vi "respond to response.vi"(8 "error in (no error)":errorcluster caption="Fehler (Eingang, kein Fehler)", 10 "?":T1={"commandlist"="", "line"=0, "last response"="", "timeout"=0, "wait"=0, "erfolgreich"=FALSE, "next state"=enum."init", "Zustand"=enum."starting", "manual Test"=FALSE}, 11 "Surge Eingang":refnum<class "Surge.lvclass"> caption="DNL_LabVIEW Object in") -> (0 "error out":errorcluster caption="Fehler (Ausgang)", 1 "read again?":bool, 2 "?":T1={"commandlist"="", "line"=0, "last response"="", "timeout"=0, "wait"=0, "erfolgreich"=FALSE, "next state"=enum."init", "Zustand"=enum."starting", "manual Test"=FALSE}, 3 "Surge Ausgang":refnum<class "Surge.lvclass"> caption="DNL_LabVIEW Object out")   [LabVIEW 2013, in "Surge.lvclass"]
uses:
  Surge.lvclass
  Main/controls/TestData.ctl
  Main/controls/TestStates.ctl
  Main/controls/generalTestStates.ctl
  lib/EMV-Test.lvlib
panel:
  out "cmdl":string
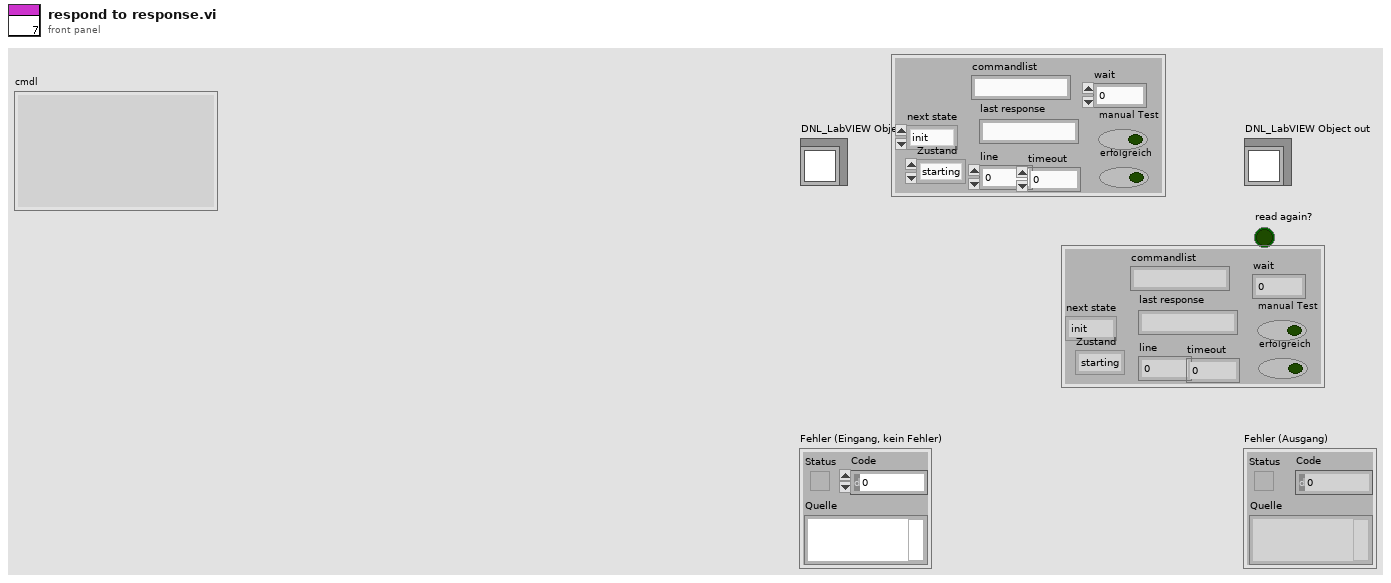
[diagram p1: front panel]
types:
  T1 = typedef "EMV-Test.lvlib/TestData.ctl" = cluster{"commandlist":string, "line":i32, "last response":string, "timeout":i32, "wait":u32, "erfolgreich":bool, "next state":T2, "Zustand":T3, "manual Test":bool}
  T2 = typedef "EMV-Test.lvlib/TestStates.ctl" = enum16{"event loop", "save Test", "Custom Action 1", "Custom Action 2", "pause", "vorgefertigter Test", "manueller Test", "respond to response", "error", "init", "start Test", "evaluate line", "wait for Response", "wait", "catch error", "close Connection", "end"}
  T3 = typedef "generalTestStates.ctl" = enum16{"paused", "starting", "waiting", "running", "finished"}
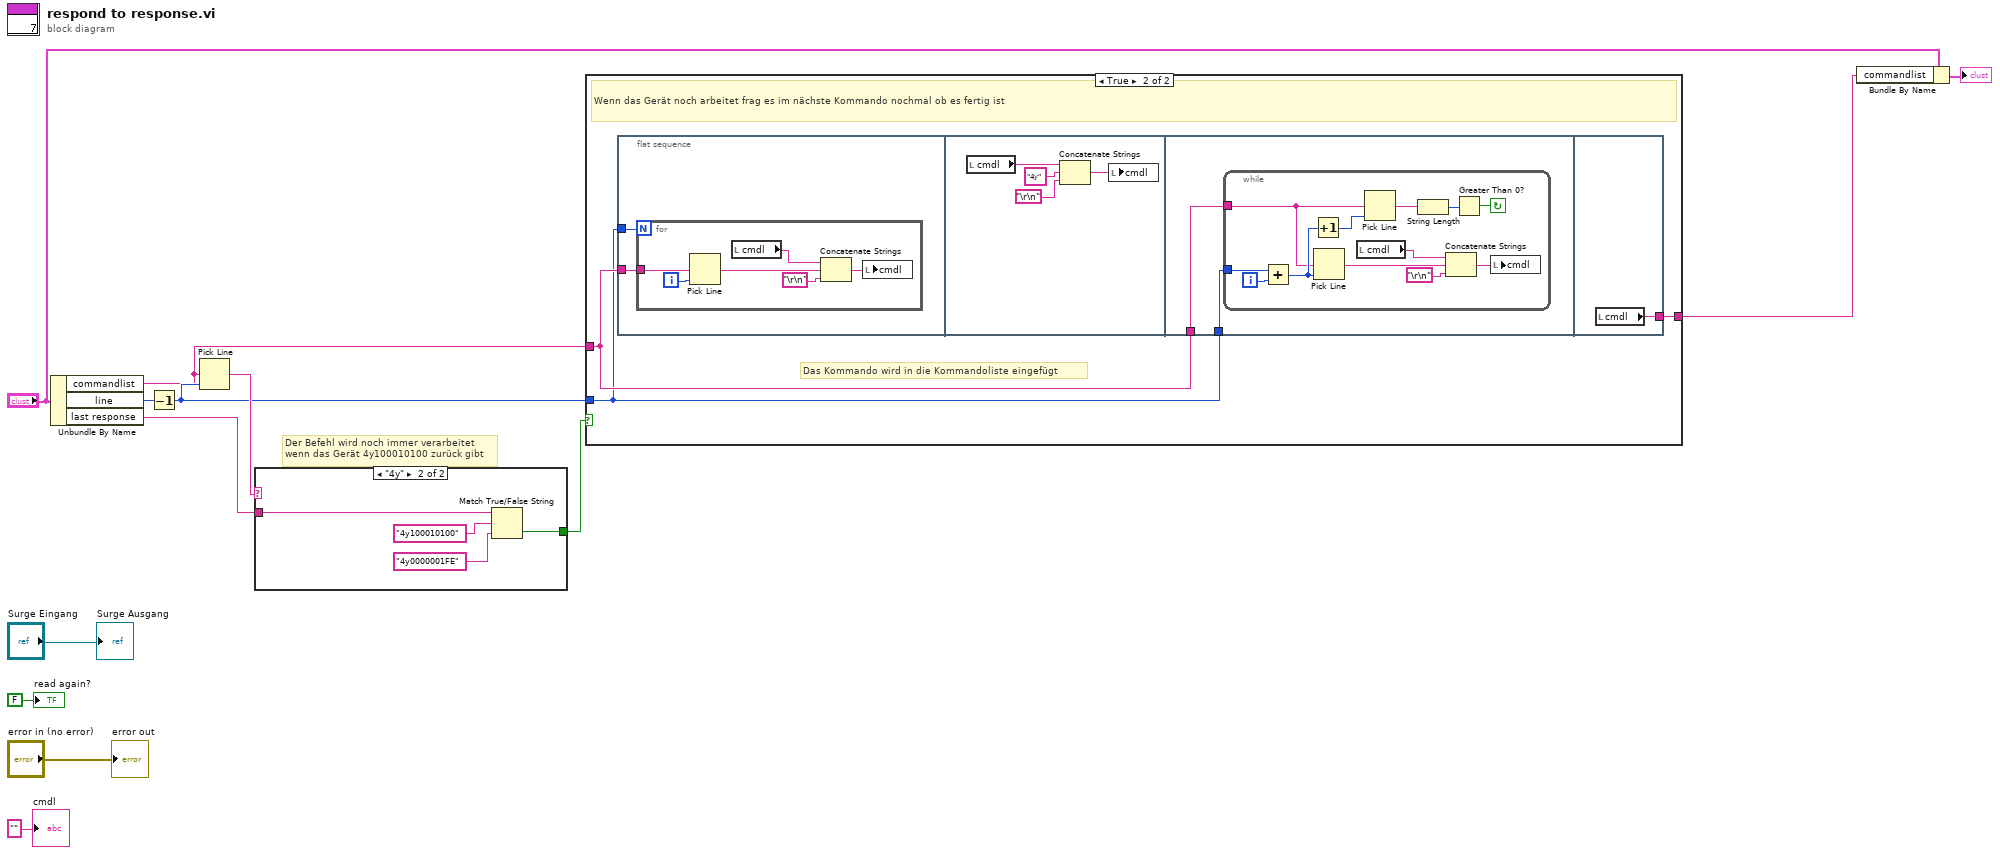
[diagram p0: block diagram]
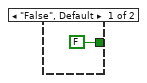
[diagram p3: hidden frame]
diagram:
  # "Der Befehl wird noch immer verarbeitet\nwenn das Gerät 4y100010100 zurück gibt"
  n1 = Unbundle By Name("?") -> ("commandlist"=w6:string, "line"=w4:i32, "last response"=w5:string)
  n2 = Decrement(x=w4) -> (x-1=w11:i32)
  n3 = Pick Line(multi-line string=w6, line index=w11) -> (output string=w13:string)  [unwired: 1 in]
  n4 = case shown="\"4y\"" w13 {
    tunnel: w5 -> [_ w18]
    tunnel: [FALSE w15] -> w12
    frame "False", Default {
    }
    frame "4y" {
      n5 = Match True/False String(2:"4y0000001FE" ("regular expression"), 3:"4y100010100" ("regular expression"), 4:w18) -> (0:w15:bool)  [unwired: 1 out]
    }
  }
  n6 = case shown="True" w12 {
    tunnel: w6 -> [w19 w22]
    tunnel: w11 -> [_ w21]
    tunnel: [w19 w20] -> w3
    frame False {
    }
    frame True {
      # "Das Kommando wird in die Kommandoliste eingefügt"
      # "Wenn das Gerät noch arbeitet frag es im nächste Kommando nochmal ob es fertig ist"
      n7 = flat-sequence {
        tunnel: w21 -> [w24]
        tunnel: w22 -> [w23]
        tunnel: w22 -> [w36]
        tunnel: w21 -> [w35]
        tunnel: [w49] -> w20
        frame #0 {
          n8 = for {
            N: w24 -> [_]
            tunnel: w23 -> [w28]
            i -> [w29]
            n9 = Pick Line(multi-line string=w28, line index=w29) -> (output string=w26:string)  [unwired: 1 in]
            n10 = local read "cmdl"() -> (w27:string)
            n11 = Concatenate Strings(w27, w26, "\r\n") -> (w30:string)
            n12 = local write "cmdl"(w30) -> ()
          }
        }
        frame #1 {
          n13 = local read "cmdl"() -> (w33:string)
          n14 = Concatenate Strings(w33, "4y" ("new Commandlist"), "\r\n") -> (w34:string)
          n15 = local write "cmdl"(w34) -> ()
        }
        frame #2 {
          n16 = while {
            tunnel: w36 -> [w44]
            tunnel: w35 -> [w47]
            i -> [w48]
            stop <- w41 continue-if-true
            n17 = Add(x=w47, y=w48) -> (x+y=w46:i32)
            n18 = Increment(x=w46) -> (x+1=w45:i32)
            n19 = Pick Line(multi-line string=w44, line index=w46) -> (output string=w38:string)  [unwired: 1 in]
            n20 = local read "cmdl"() -> (w39:string)
            n21 = Pick Line(multi-line string=w44, line index=w45) -> (output string=w43:string)  [unwired: 1 in]
            n22 = String Length(string=w43) -> (length=w42:i32)
            n23 = Concatenate Strings(w39, w38, "\r\n") -> (w40:string)
            n24 = Greater Than 0?(x=w42) -> (x > 0?=w41:bool)
            n25 = local write "cmdl"(w40) -> ()
          }
        }
        frame #3 {
          n26 = local read "cmdl"() -> (w49:string)
        }
      }
    }
  }
  n27 = Bundle By Name(cluster="?", "commandlist"=w3) -> (→"?":T1)
  "error out" <- "error in (no error)"
  "Surge Ausgang" <- "Surge Eingang"
  "read again?" <- FALSE ("read again?")
  "cmdl" <- ""
